vi "SetLogFormatter.vi"(8 "Error in (no error)":errorcluster, 10 "LogFormatterInterface in":refnum<class "LogFormatterInterface.lvclass">, 11 "LogWriterMock in":refnum<class "LogWriterMock.lvclass">) -> (0 "Error out":errorcluster, 3 "LogWriterMock out":refnum<class "LogWriterMock.lvclass">)   [LabVIEW 2011, in "LogWriterMock.lvclass"]
uses:
  LogWriterMock.lvclass
  Formatter/LogFormatterInterface/LogFormatterInterface.lvclass
  LogWriterInterface/LogWriterInterface.lvclass
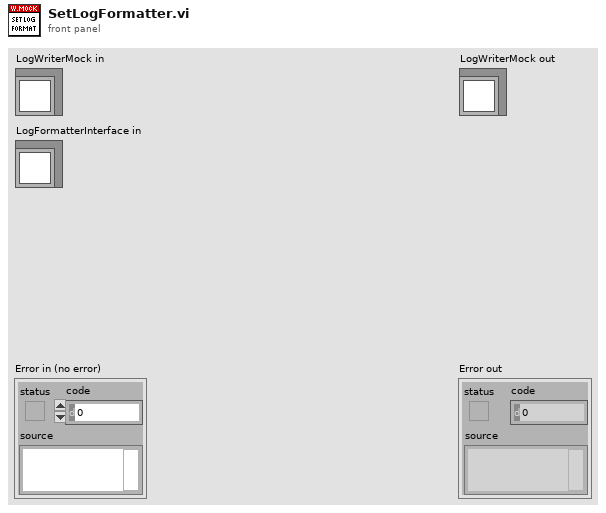
[diagram p1: front panel]
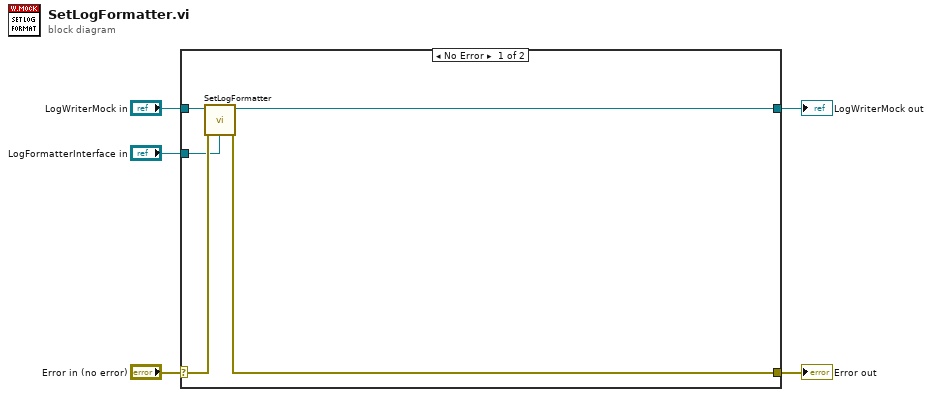
[diagram p0: block diagram]
diagram:
  n1 = case shown="No Error" "Error in (no error)" {
    selector: "Error in (no error)" -> [w8 w12]
    tunnel: [w7 w12] -> w4
    tunnel: [w9 w11] -> w2
    tunnel: "LogWriterMock in" -> [w10 w11]
    tunnel: "LogFormatterInterface in" -> [w6 _]
    frame No Error {
      n2 = call-parent "SetLogFormatter.vi"("Error in (no error)"=w8, "LogFormatterInterface in"=w6, "LogWriterInterface in"=w10) -> ("Error out"=w7:errorcluster, "LogWriterInterface out"=w9:refnum<class "LogWriterMock.lvclass">)  [unwired: 7 in]
    }
    frame Error {
    }
  }
  "Error out" <- w4
  "LogWriterMock out" <- w2
